vi "InitDrivebase.vi"   [LabVIEW 2020]
doc: "This VI initializes devices related directly to the drive subsystem."
uses:
  <vilib>/Rock Robotics/WPI/Solenoid/WPI_SolenoidChannel.ctl
  <vilib>/Rock Robotics/WPI/ThirdParty/Phoenix-LabVIEW/Motor Controller/Controls/CTRE_Phoenix_MotorControl_NeutralMode.ctl
  <vilib>/Rock Robotics/WPI/ThirdParty/Phoenix-LabVIEW/Motor Controller/Controls/CTRE_Phoenix_MotorControl_SupplyCurrentLimitConfiguration.ctl
  <vilib>/Rock Robotics/WPI/ThirdParty/Phoenix-LabVIEW/Motor Controller/Controls/CTRE_Phoenix_MotorControl_FeedbackDevice_TalonFX.ctl
  <vilib>/Rock Robotics/WPI/ThirdParty/Phoenix-LabVIEW/Motor Controller/Controls/CTRE_Phoenix_MotorControl_TalonFXInvertType.ctl
  <vilib>/Rock Robotics/WPI/Solenoid/WPI_SolenoidOpenDouble.vi
  refnums.vi
types:
  T1 = typedef "WPI_SolenoidChannel.ctl" = enum8{"Solenoid 0", "Solenoid 1", "Solenoid 2", "Solenoid 3", "Solenoid 4", "Solenoid 5", "Solenoid 6", "Solenoid 7", "Solenoid 8", "Solenoid 9", "Solenoid 10", "Solenoid 11", "Solenoid 12", "Solenoid 13", "Solenoid 14", "Solenoid 15", "Invalid"}
  T2 = typedef "CTRE_Phoenix_MotorControl_TalonFXInvertType.ctl" = enum16{"Counter-Clockwise", "Clockwise"}
  T3 = typedef "CTRE_Phoenix_MotorControl_FeedbackDevice_TalonFX.ctl" = i8
  T4 = typedef "CTRE_Phoenix_MotorControl_SupplyCurrentLimitConfiguration.ctl" = cluster{"Enable?":bool, "Current Limit":dbl, "Threshold Current":dbl, "Threshold Time":dbl}
  T5 = typedef "CTRE_Phoenix_MotorControl_NeutralMode.ctl" = enum8{"EEPROMSetting", "Override to Coast", "Override to Brake"}
  T6 = typedef "WPI_MotorControlDeviceRef.ctl" = cluster{"DeviceStatus":errorcluster, "Type":T7, "PWM":cluster{"PWM Channel":T8, "DeadBand":T9}, "CAN":cluster{"Device Number":u8, "SetOutput VI Ref":variant, "GetOutput VI Ref":variant, "Enable VI Ref":variant, "Disable VI Ref":variant, "Data":variant}, "Invert":bool, "DIO PWM":cluster{"PWM \"Enable\" Channel":T8, "DIOChannel":T10, "PWM Rate":dbl}}
  T7 = typedef "WPI_MotorControlType.ctl" = enum16{"PWM", "CAN", "DIO PWM"}
  T8 = typedef "FPGA_DIOPWMChannel.ctl" = enum8{"PWM 0", "PWM 1", "PWM 2", "PWM 3", "PWM 4", "PWM 5", "PWM 6", "PWM 7", "PWM 8", "PWM 9", "PWM MXP 0", "PWM MXP 1", "PWM MXP 2", "PWM MXP 3", "PWM MXP 4", "PWM MXP 5", "PWM MXP 6", "PWM MXP 7", "PWM MXP 8", "PWM MXP 9", "Invalid"}
  T9 = typedef "WPI_PWMDeadband.ctl" = cluster{"Name":string, "maxPositivePwm":i32, "minPositivePwm":i32, "centerPwm":i32, "maxNegativePwm":i32, "minNegativePwm":i32, "angularRange":u16}
  T10 = typedef "FPGA_DIOChannel.ctl" = enum8{"DIO 0", "DIO 1", "DIO 2", "DIO 3", "DIO 4", "DIO 5", "DIO 6", "DIO 7", "DIO 8", "DIO 9", "DIO MXP 0", "DIO MXP 1", "DIO MXP 2", "DIO MXP 3", "DIO MXP 4", "DIO MXP 5", "DIO MXP 6", "DIO MXP 7", "DIO MXP 8", "DIO MXP 9", "DIO MXP 10", "DIO MXP 11", "DIO MXP 12", "DIO MXP 13", "DIO MXP 14", "DIO MXP 15", "SPI Port CS1", "SPI Port CS2", "SPI Port CS3", "SPI Port MISO", "SPI Port MOSI", "Invalid"}
  T11 = typedef "WPI_SolenoidDevRef.ctl" = cluster{"DevStatus":errorcluster, "Pneumatics Control Module":u8, "Forward Solenoid Channel":T1, "Reverse Solenoid Channel":T1}
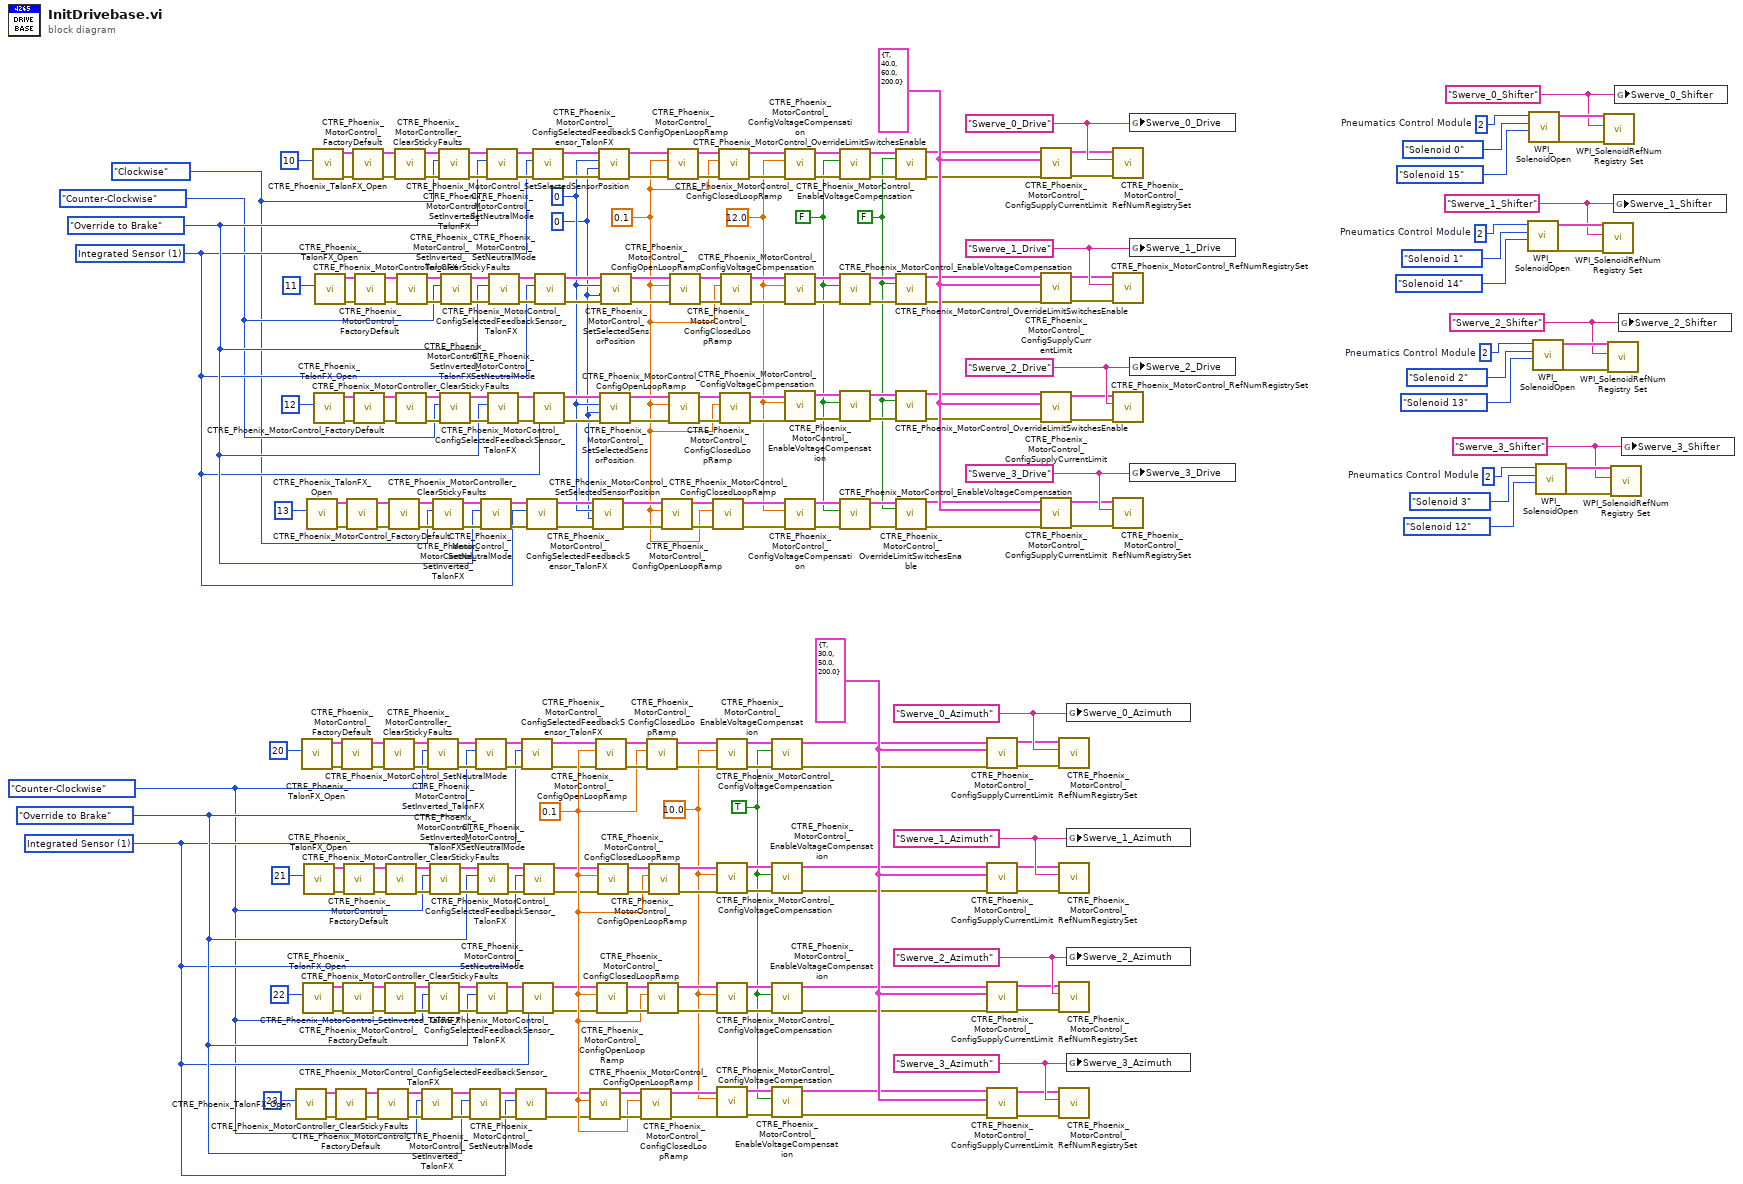
[diagram p0: block diagram]
diagram:
  w9 = FALSE ("Override Limit Switch Enable?")
  w27 = "Swerve_0_Shifter" ("refnum name")
  w32 = u8 2  # Pneumatics Control Module
  w33 = "Swerve_1_Shifter" ("refnum name")
  w38 = u8 2  # Pneumatics Control Module
  w39 = "Swerve_2_Shifter" ("refnum name")
  w44 = u8 2  # Pneumatics Control Module
  w45 = CTRE_Phoenix_MotorControl_TalonFXInvertType."Clockwise" ("Invert Type")
  w47 = TRUE ("Enable Voltage Compensation?")
  w48 = 10.0 ("Saturation Voltage")
  w49 = FALSE ("Enable Voltage Compensation?")
  w50 = 12.0 ("Saturation Voltage")
  w91 = T3 1 items=["Integrated Sensor"=1, "Sensor Sum (S0 + S1)"=9, "Sensor Difference (D0 - D1)"=10, "Remote Source 0"=11, "Remote Source 1"=12, "None"=14, "Software Emulated"=15] ("Talon FX Feedback Device")
  w94 = T4 {"Enable?"=TRUE, "Current Limit"=30.0, "Threshold Current"=50.0, "Threshold Time"=200.0} ("Supply Current Limit Configuration")
  w92 = 0.1 ("secondsFromNeutralToFull")
  w93 = CTRE_Phoenix_MotorControl_NeutralMode."Override to Brake" ("Motor Control Neutral Mode")
  w26 = CTRE_Phoenix_MotorControl_TalonFXInvertType."Counter-Clockwise" ("Invert Type")
  w108 = "Swerve_0_Azimuth" ("refnum name")
  w124 = "Swerve_1_Azimuth" ("refnum name")
  w140 = "Swerve_2_Azimuth" ("refnum name")
  w156 = "Swerve_3_Azimuth" ("refnum name")
  w162 = T3 1 items=["Integrated Sensor"=1, "Sensor Sum (S0 + S1)"=9, "Sensor Difference (D0 - D1)"=10, "Remote Source 0"=11, "Remote Source 1"=12, "None"=14, "Software Emulated"=15] ("Talon FX Feedback Device")
  w164 = T4 {"Enable?"=TRUE, "Current Limit"=40.0, "Threshold Current"=60.0, "Threshold Time"=200.0} ("Supply Current Limit Configuration")
  w159 = 0.1 ("secondsFromNeutralToFull")
  w160 = u32 0 ("pidLoopIdx")
  w161 = 0 ("New Sensor Position")
  w163 = CTRE_Phoenix_MotorControl_NeutralMode."Override to Brake" ("Motor Control Neutral Mode")
  w46 = CTRE_Phoenix_MotorControl_TalonFXInvertType."Counter-Clockwise" ("Invert Type")
  w180 = "Swerve_0_Drive" ("refnum name")
  w200 = "Swerve_1_Drive" ("refnum name")
  w220 = "Swerve_2_Drive" ("refnum name")
  w240 = "Swerve_3_Drive" ("refnum name")
  w245 = "Swerve_3_Shifter" ("refnum name")
  w250 = u8 2  # Pneumatics Control Module
  n1 = call <vilib>:"CTRE_Phoenix_TalonFX_Open.vi"("Device Number"=u8 23 ("Drive 4L")) -> ("error out"=w145:errorcluster, "PhoenixMotorControlDevRef"=w152:T6)  [unwired: 9 in]
  n2 = call <vilib>:"CTRE_Phoenix_TalonFX_Open.vi"("Device Number"=u8 20 ("Drive 4L")) -> ("error out"=w97:errorcluster, "PhoenixMotorControlDevRef"=w104:T6)  [unwired: 9 in]
  n3 = call <vilib>:"CTRE_Phoenix_TalonFX_Open.vi"("Device Number"=u8 22 ("Drive 4L")) -> ("error out"=w129:errorcluster, "PhoenixMotorControlDevRef"=w136:T6)  [unwired: 9 in]
  n4 = call <vilib>:"CTRE_Phoenix_TalonFX_Open.vi"("Device Number"=u8 21 ("Drive 4L")) -> ("error out"=w113:errorcluster, "PhoenixMotorControlDevRef"=w120:T6)  [unwired: 9 in]
  n5 = call <vilib>:"CTRE_Phoenix_TalonFX_Open.vi"("Device Number"=u8 13 ("Drive 4L")) -> ("error out"=w229:errorcluster, "PhoenixMotorControlDevRef"=w236:T6)  [unwired: 9 in]
  n6 = call <vilib>:"CTRE_Phoenix_TalonFX_Open.vi"("Device Number"=u8 10 ("Drive 4L")) -> ("error out"=w169:errorcluster, "PhoenixMotorControlDevRef"=w176:T6)  [unwired: 9 in]
  n7 = call <vilib>:"CTRE_Phoenix_TalonFX_Open.vi"("Device Number"=u8 12 ("Drive 4L")) -> ("error out"=w209:errorcluster, "PhoenixMotorControlDevRef"=w216:T6)  [unwired: 9 in]
  n8 = call <vilib>:"CTRE_Phoenix_TalonFX_Open.vi"("Device Number"=u8 11 ("Drive 4L")) -> ("error out"=w189:errorcluster, "PhoenixMotorControlDevRef"=w196:T6)  [unwired: 9 in]
  n9 = call <vilib>:"CTRE_Phoenix_MotorControl_FactoryDefault.vi"("error in"=w145, "PhoenixMotorControlDevRef"=w152) -> ("error out"=w148:errorcluster, "PhoenixMotorControlDevRef"=w149:T6)  [unwired: 8 in]
  n10 = call <vilib>:"CTRE_Phoenix_MotorControl_FactoryDefault.vi"("error in"=w97, "PhoenixMotorControlDevRef"=w104) -> ("error out"=w100:errorcluster, "PhoenixMotorControlDevRef"=w101:T6)  [unwired: 8 in]
  n11 = call <vilib>:"CTRE_Phoenix_MotorControl_FactoryDefault.vi"("error in"=w129, "PhoenixMotorControlDevRef"=w136) -> ("error out"=w132:errorcluster, "PhoenixMotorControlDevRef"=w133:T6)  [unwired: 8 in]
  n12 = call <vilib>:"CTRE_Phoenix_MotorControl_FactoryDefault.vi"("error in"=w113, "PhoenixMotorControlDevRef"=w120) -> ("error out"=w116:errorcluster, "PhoenixMotorControlDevRef"=w117:T6)  [unwired: 8 in]
  n13 = call <vilib>:"CTRE_Phoenix_MotorControl_FactoryDefault.vi"("error in"=w229, "PhoenixMotorControlDevRef"=w236) -> ("error out"=w232:errorcluster, "PhoenixMotorControlDevRef"=w233:T6)  [unwired: 8 in]
  n14 = call <vilib>:"CTRE_Phoenix_MotorControl_FactoryDefault.vi"("error in"=w169, "PhoenixMotorControlDevRef"=w176) -> ("error out"=w172:errorcluster, "PhoenixMotorControlDevRef"=w173:T6)  [unwired: 8 in]
  n15 = call <vilib>:"CTRE_Phoenix_MotorControl_FactoryDefault.vi"("error in"=w209, "PhoenixMotorControlDevRef"=w216) -> ("error out"=w212:errorcluster, "PhoenixMotorControlDevRef"=w213:T6)  [unwired: 8 in]
  n16 = call <vilib>:"CTRE_Phoenix_MotorControl_FactoryDefault.vi"("error in"=w189, "PhoenixMotorControlDevRef"=w196) -> ("error out"=w192:errorcluster, "PhoenixMotorControlDevRef"=w193:T6)  [unwired: 8 in]
  n17 = call <vilib>:"CTRE_Phoenix_MotorController_ClearStickyFaults.vi"("error in"=w148, "PhoenixMotorControlDevRef"=w149) -> ("error out"=w147:errorcluster, "PhoenixMotorControlDevRef"=w146:T6)  [unwired: 8 in]
  n18 = call <vilib>:"CTRE_Phoenix_MotorController_ClearStickyFaults.vi"("error in"=w100, "PhoenixMotorControlDevRef"=w101) -> ("error out"=w99:errorcluster, "PhoenixMotorControlDevRef"=w98:T6)  [unwired: 8 in]
  n19 = call <vilib>:"CTRE_Phoenix_MotorController_ClearStickyFaults.vi"("error in"=w132, "PhoenixMotorControlDevRef"=w133) -> ("error out"=w131:errorcluster, "PhoenixMotorControlDevRef"=w130:T6)  [unwired: 8 in]
  n20 = call <vilib>:"CTRE_Phoenix_MotorController_ClearStickyFaults.vi"("error in"=w116, "PhoenixMotorControlDevRef"=w117) -> ("error out"=w115:errorcluster, "PhoenixMotorControlDevRef"=w114:T6)  [unwired: 8 in]
  n21 = call <vilib>:"CTRE_Phoenix_MotorController_ClearStickyFaults.vi"("error in"=w232, "PhoenixMotorControlDevRef"=w233) -> ("error out"=w231:errorcluster, "PhoenixMotorControlDevRef"=w230:T6)  [unwired: 8 in]
  n22 = call <vilib>:"CTRE_Phoenix_MotorController_ClearStickyFaults.vi"("error in"=w172, "PhoenixMotorControlDevRef"=w173) -> ("error out"=w171:errorcluster, "PhoenixMotorControlDevRef"=w170:T6)  [unwired: 8 in]
  n23 = call <vilib>:"CTRE_Phoenix_MotorController_ClearStickyFaults.vi"("error in"=w212, "PhoenixMotorControlDevRef"=w213) -> ("error out"=w211:errorcluster, "PhoenixMotorControlDevRef"=w210:T6)  [unwired: 8 in]
  n24 = call <vilib>:"CTRE_Phoenix_MotorController_ClearStickyFaults.vi"("error in"=w192, "PhoenixMotorControlDevRef"=w193) -> ("error out"=w191:errorcluster, "PhoenixMotorControlDevRef"=w190:T6)  [unwired: 8 in]
  n25 = call <vilib>:"CTRE_Phoenix_MotorControl_SetInverted_TalonFX.vi"("error in (no error)"=w147, "Invert Type"=w26, "PhoenixMotorControlDevRef"=w146) -> ("error out"=w157:errorcluster, "PhoenixMotorControlDevRef"=w158:T6)  [unwired: 7 in]
  n26 = call <vilib>:"CTRE_Phoenix_MotorControl_SetInverted_TalonFX.vi"("error in (no error)"=w99, "Invert Type"=w26, "PhoenixMotorControlDevRef"=w98) -> ("error out"=w109:errorcluster, "PhoenixMotorControlDevRef"=w110:T6)  [unwired: 7 in]
  n27 = call <vilib>:"CTRE_Phoenix_MotorControl_SetInverted_TalonFX.vi"("error in (no error)"=w131, "Invert Type"=w26, "PhoenixMotorControlDevRef"=w130) -> ("error out"=w141:errorcluster, "PhoenixMotorControlDevRef"=w142:T6)  [unwired: 7 in]
  n28 = call <vilib>:"CTRE_Phoenix_MotorControl_SetInverted_TalonFX.vi"("error in (no error)"=w115, "Invert Type"=w26, "PhoenixMotorControlDevRef"=w114) -> ("error out"=w125:errorcluster, "PhoenixMotorControlDevRef"=w126:T6)  [unwired: 7 in]
  n29 = call <vilib>:"CTRE_Phoenix_MotorControl_SetInverted_TalonFX.vi"("error in (no error)"=w231, "Invert Type"=w45, "PhoenixMotorControlDevRef"=w230) -> ("error out"=w243:errorcluster, "PhoenixMotorControlDevRef"=w244:T6)  [unwired: 7 in]
  n30 = call <vilib>:"CTRE_Phoenix_MotorControl_SetInverted_TalonFX.vi"("error in (no error)"=w171, "Invert Type"=w45, "PhoenixMotorControlDevRef"=w170) -> ("error out"=w183:errorcluster, "PhoenixMotorControlDevRef"=w184:T6)  [unwired: 7 in]
  n31 = call <vilib>:"CTRE_Phoenix_MotorControl_SetInverted_TalonFX.vi"("error in (no error)"=w211, "Invert Type"=w46, "PhoenixMotorControlDevRef"=w210) -> ("error out"=w223:errorcluster, "PhoenixMotorControlDevRef"=w224:T6)  [unwired: 7 in]
  n32 = call <vilib>:"CTRE_Phoenix_MotorControl_SetInverted_TalonFX.vi"("error in (no error)"=w191, "Invert Type"=w46, "PhoenixMotorControlDevRef"=w190) -> ("error out"=w203:errorcluster, "PhoenixMotorControlDevRef"=w204:T6)  [unwired: 7 in]
  n33 = call <vilib>:"CTRE_Phoenix_MotorControl_SetNeutralMode.vi"("error in (no error)"=w157, "Motor Control Neutral Mode"=w93, "PhoenixMotorControlDevRef"=w158) -> ("error out"=w143:errorcluster, "PhoenixMotorControlDevRef"=w144:T6)  [unwired: 7 in]
  n34 = call <vilib>:"CTRE_Phoenix_MotorControl_SetNeutralMode.vi"("error in (no error)"=w109, "Motor Control Neutral Mode"=w93, "PhoenixMotorControlDevRef"=w110) -> ("error out"=w95:errorcluster, "PhoenixMotorControlDevRef"=w96:T6)  [unwired: 7 in]
  n35 = call <vilib>:"CTRE_Phoenix_MotorControl_SetNeutralMode.vi"("error in (no error)"=w141, "Motor Control Neutral Mode"=w93, "PhoenixMotorControlDevRef"=w142) -> ("error out"=w127:errorcluster, "PhoenixMotorControlDevRef"=w128:T6)  [unwired: 7 in]
  n36 = call <vilib>:"CTRE_Phoenix_MotorControl_SetNeutralMode.vi"("error in (no error)"=w125, "Motor Control Neutral Mode"=w93, "PhoenixMotorControlDevRef"=w126) -> ("error out"=w111:errorcluster, "PhoenixMotorControlDevRef"=w112:T6)  [unwired: 7 in]
  n37 = call <vilib>:"CTRE_Phoenix_MotorControl_SetNeutralMode.vi"("error in (no error)"=w243, "Motor Control Neutral Mode"=w163, "PhoenixMotorControlDevRef"=w244) -> ("error out"=w227:errorcluster, "PhoenixMotorControlDevRef"=w228:T6)  [unwired: 7 in]
  n38 = call <vilib>:"CTRE_Phoenix_MotorControl_SetNeutralMode.vi"("error in (no error)"=w183, "Motor Control Neutral Mode"=w163, "PhoenixMotorControlDevRef"=w184) -> ("error out"=w167:errorcluster, "PhoenixMotorControlDevRef"=w168:T6)  [unwired: 7 in]
  n39 = call <vilib>:"CTRE_Phoenix_MotorControl_SetNeutralMode.vi"("error in (no error)"=w223, "Motor Control Neutral Mode"=w163, "PhoenixMotorControlDevRef"=w224) -> ("error out"=w207:errorcluster, "PhoenixMotorControlDevRef"=w208:T6)  [unwired: 7 in]
  n40 = call <vilib>:"CTRE_Phoenix_MotorControl_SetNeutralMode.vi"("error in (no error)"=w203, "Motor Control Neutral Mode"=w163, "PhoenixMotorControlDevRef"=w204) -> ("error out"=w187:errorcluster, "PhoenixMotorControlDevRef"=w188:T6)  [unwired: 7 in]
  n41 = call <vilib>:"CTRE_Phoenix_MotorControl_ConfigSelectedFeedbackSensor_TalonFX.vi"("error in (no error)"=w143, "Talon FX Feedback Device"=w91, "PhoenixMotorControlDevRef"=w144) -> ("error out"=w7:errorcluster, "PhoenixMotorControlDevRef"=w8:T6)  [unwired: 7 in]
  n42 = call <vilib>:"CTRE_Phoenix_MotorControl_ConfigSelectedFeedbackSensor_TalonFX.vi"("error in (no error)"=w95, "Talon FX Feedback Device"=w91, "PhoenixMotorControlDevRef"=w96) -> ("error out"=w1:errorcluster, "PhoenixMotorControlDevRef"=w2:T6)  [unwired: 7 in]
  n43 = call <vilib>:"CTRE_Phoenix_MotorControl_ConfigSelectedFeedbackSensor_TalonFX.vi"("error in (no error)"=w127, "Talon FX Feedback Device"=w91, "PhoenixMotorControlDevRef"=w128) -> ("error out"=w5:errorcluster, "PhoenixMotorControlDevRef"=w6:T6)  [unwired: 7 in]
  n44 = call <vilib>:"CTRE_Phoenix_MotorControl_ConfigSelectedFeedbackSensor_TalonFX.vi"("error in (no error)"=w111, "Talon FX Feedback Device"=w91, "PhoenixMotorControlDevRef"=w112) -> ("error out"=w3:errorcluster, "PhoenixMotorControlDevRef"=w4:T6)  [unwired: 7 in]
  n45 = call <vilib>:"CTRE_Phoenix_MotorControl_ConfigSelectedFeedbackSensor_TalonFX.vi"("error in (no error)"=w227, "Talon FX Feedback Device"=w162, "PhoenixMotorControlDevRef"=w228) -> ("error out"=w225:errorcluster, "PhoenixMotorControlDevRef"=w226:T6)  [unwired: 7 in]
  n46 = call <vilib>:"CTRE_Phoenix_MotorControl_ConfigSelectedFeedbackSensor_TalonFX.vi"("error in (no error)"=w167, "Talon FX Feedback Device"=w162, "PhoenixMotorControlDevRef"=w168) -> ("error out"=w165:errorcluster, "PhoenixMotorControlDevRef"=w166:T6)  [unwired: 7 in]
  n47 = call <vilib>:"CTRE_Phoenix_MotorControl_ConfigSelectedFeedbackSensor_TalonFX.vi"("error in (no error)"=w207, "Talon FX Feedback Device"=w162, "PhoenixMotorControlDevRef"=w208) -> ("error out"=w205:errorcluster, "PhoenixMotorControlDevRef"=w206:T6)  [unwired: 7 in]
  n48 = call <vilib>:"CTRE_Phoenix_MotorControl_ConfigSelectedFeedbackSensor_TalonFX.vi"("error in (no error)"=w187, "Talon FX Feedback Device"=w162, "PhoenixMotorControlDevRef"=w188) -> ("error out"=w185:errorcluster, "PhoenixMotorControlDevRef"=w186:T6)  [unwired: 7 in]
  n49 = call <vilib>:"CTRE_Phoenix_MotorControl_ConfigOpenLoopRamp.vi"("error in (no error)"=w7, "secondsFromNeutralToFull"=w92, "PhoenixMotorControlDevRef"=w8) -> ("error out"=w150:errorcluster, "PhoenixMotorControlDevRef"=w151:T6)  [unwired: 7 in]
  n50 = call <vilib>:"CTRE_Phoenix_MotorControl_SetSelectedSensorPosition.vi"("error in (no error)"=w225, "pidLoopIdx"=w160, "New Sensor Position"=w161, "PhoenixMotorControlDevRef"=w226) -> ("error out"=w242:errorcluster, "PhoenixMotorControlDevRef"=w241:T6)  [unwired: 6 in]
  n51 = call <vilib>:"CTRE_Phoenix_MotorControl_ConfigOpenLoopRamp.vi"("error in (no error)"=w1, "secondsFromNeutralToFull"=w92, "PhoenixMotorControlDevRef"=w2) -> ("error out"=w102:errorcluster, "PhoenixMotorControlDevRef"=w103:T6)  [unwired: 7 in]
  n52 = call <vilib>:"CTRE_Phoenix_MotorControl_ConfigOpenLoopRamp.vi"("error in (no error)"=w5, "secondsFromNeutralToFull"=w92, "PhoenixMotorControlDevRef"=w6) -> ("error out"=w134:errorcluster, "PhoenixMotorControlDevRef"=w135:T6)  [unwired: 7 in]
  n53 = call <vilib>:"CTRE_Phoenix_MotorControl_ConfigOpenLoopRamp.vi"("error in (no error)"=w3, "secondsFromNeutralToFull"=w92, "PhoenixMotorControlDevRef"=w4) -> ("error out"=w118:errorcluster, "PhoenixMotorControlDevRef"=w119:T6)  [unwired: 7 in]
  n54 = call <vilib>:"CTRE_Phoenix_MotorControl_SetSelectedSensorPosition.vi"("error in (no error)"=w165, "pidLoopIdx"=w160, "New Sensor Position"=w161, "PhoenixMotorControlDevRef"=w166) -> ("error out"=w182:errorcluster, "PhoenixMotorControlDevRef"=w181:T6)  [unwired: 6 in]
  n55 = call <vilib>:"CTRE_Phoenix_MotorControl_SetSelectedSensorPosition.vi"("error in (no error)"=w205, "pidLoopIdx"=w160, "New Sensor Position"=w161, "PhoenixMotorControlDevRef"=w206) -> ("error out"=w222:errorcluster, "PhoenixMotorControlDevRef"=w221:T6)  [unwired: 6 in]
  n56 = call <vilib>:"CTRE_Phoenix_MotorControl_SetSelectedSensorPosition.vi"("error in (no error)"=w185, "pidLoopIdx"=w160, "New Sensor Position"=w161, "PhoenixMotorControlDevRef"=w186) -> ("error out"=w202:errorcluster, "PhoenixMotorControlDevRef"=w201:T6)  [unwired: 6 in]
  n57 = call <vilib>:"CTRE_Phoenix_MotorControl_ConfigClosedLoopRamp.vi"("error in (no error)"=w150, "secondsFromNeutralToFull"=w92, "PhoenixMotorControlDevRef"=w151) -> ("error out"=w53:errorcluster, "PhoenixMotorControlDevRef"=w54:T6)  [unwired: 7 in]
  n58 = call <vilib>:"CTRE_Phoenix_MotorControl_ConfigClosedLoopRamp.vi"("error in (no error)"=w102, "secondsFromNeutralToFull"=w92, "PhoenixMotorControlDevRef"=w103) -> ("error out"=w65:errorcluster, "PhoenixMotorControlDevRef"=w66:T6)  [unwired: 7 in]
  n59 = call <vilib>:"CTRE_Phoenix_MotorControl_ConfigClosedLoopRamp.vi"("error in (no error)"=w134, "secondsFromNeutralToFull"=w92, "PhoenixMotorControlDevRef"=w135) -> ("error out"=w57:errorcluster, "PhoenixMotorControlDevRef"=w58:T6)  [unwired: 7 in]
  n60 = call <vilib>:"CTRE_Phoenix_MotorControl_ConfigClosedLoopRamp.vi"("error in (no error)"=w118, "secondsFromNeutralToFull"=w92, "PhoenixMotorControlDevRef"=w119) -> ("error out"=w61:errorcluster, "PhoenixMotorControlDevRef"=w62:T6)  [unwired: 7 in]
  n61 = call <vilib>:"CTRE_Phoenix_MotorControl_ConfigOpenLoopRamp.vi"("error in (no error)"=w242, "secondsFromNeutralToFull"=w159, "PhoenixMotorControlDevRef"=w241) -> ("error out"=w234:errorcluster, "PhoenixMotorControlDevRef"=w235:T6)  [unwired: 7 in]
  n62 = call <vilib>:"CTRE_Phoenix_MotorControl_ConfigOpenLoopRamp.vi"("error in (no error)"=w182, "secondsFromNeutralToFull"=w159, "PhoenixMotorControlDevRef"=w181) -> ("error out"=w174:errorcluster, "PhoenixMotorControlDevRef"=w175:T6)  [unwired: 7 in]
  n63 = call <vilib>:"CTRE_Phoenix_MotorControl_ConfigOpenLoopRamp.vi"("error in (no error)"=w222, "secondsFromNeutralToFull"=w159, "PhoenixMotorControlDevRef"=w221) -> ("error out"=w214:errorcluster, "PhoenixMotorControlDevRef"=w215:T6)  [unwired: 7 in]
  n64 = call <vilib>:"CTRE_Phoenix_MotorControl_ConfigOpenLoopRamp.vi"("error in (no error)"=w202, "secondsFromNeutralToFull"=w159, "PhoenixMotorControlDevRef"=w201) -> ("error out"=w194:errorcluster, "PhoenixMotorControlDevRef"=w195:T6)  [unwired: 7 in]
  n65 = call <vilib>:"CTRE_Phoenix_MotorControl_ConfigClosedLoopRamp.vi"("error in (no error)"=w234, "secondsFromNeutralToFull"=w159, "PhoenixMotorControlDevRef"=w235) -> ("error out"=w67:errorcluster, "PhoenixMotorControlDevRef"=w68:T6)  [unwired: 7 in]
  n66 = call <vilib>:"CTRE_Phoenix_MotorControl_ConfigVoltageCompensation.vi"("error in (no error)"=w65, "Saturation Voltage"=w48, "PhoenixMotorControlDevRef"=w66) -> ("error out"=w81:errorcluster, "PhoenixMotorControlDevRef"=w82:T6)  [unwired: 7 in]
  n67 = call <vilib>:"CTRE_Phoenix_MotorControl_ConfigVoltageCompensation.vi"("error in (no error)"=w61, "Saturation Voltage"=w48, "PhoenixMotorControlDevRef"=w62) -> ("error out"=w79:errorcluster, "PhoenixMotorControlDevRef"=w80:T6)  [unwired: 7 in]
  n68 = call <vilib>:"CTRE_Phoenix_MotorControl_ConfigVoltageCompensation.vi"("error in (no error)"=w57, "Saturation Voltage"=w48, "PhoenixMotorControlDevRef"=w58) -> ("error out"=w77:errorcluster, "PhoenixMotorControlDevRef"=w78:T6)  [unwired: 7 in]
  n69 = call <vilib>:"CTRE_Phoenix_MotorControl_ConfigVoltageCompensation.vi"("error in (no error)"=w53, "Saturation Voltage"=w48, "PhoenixMotorControlDevRef"=w54) -> ("error out"=w75:errorcluster, "PhoenixMotorControlDevRef"=w76:T6)  [unwired: 7 in]
  n70 = call <vilib>:"CTRE_Phoenix_MotorControl_ConfigClosedLoopRamp.vi"("error in (no error)"=w174, "secondsFromNeutralToFull"=w159, "PhoenixMotorControlDevRef"=w175) -> ("error out"=w73:errorcluster, "PhoenixMotorControlDevRef"=w74:T6)  [unwired: 7 in]
  n71 = call <vilib>:"CTRE_Phoenix_MotorControl_ConfigClosedLoopRamp.vi"("error in (no error)"=w214, "secondsFromNeutralToFull"=w159, "PhoenixMotorControlDevRef"=w215) -> ("error out"=w69:errorcluster, "PhoenixMotorControlDevRef"=w70:T6)  [unwired: 7 in]
  n72 = call <vilib>:"CTRE_Phoenix_MotorControl_ConfigClosedLoopRamp.vi"("error in (no error)"=w194, "secondsFromNeutralToFull"=w159, "PhoenixMotorControlDevRef"=w195) -> ("error out"=w71:errorcluster, "PhoenixMotorControlDevRef"=w72:T6)  [unwired: 7 in]
  n73 = call <vilib>:"CTRE_Phoenix_MotorControl_EnableVoltageCompensation.vi"("error in (no error)"=w81, "Enable Voltage Compensation?"=w47, "PhoenixMotorControlDevRef"=w82) -> ("error out"=w63:errorcluster, "PhoenixMotorControlDevRef"=w64:T6)  [unwired: 7 in]
  n74 = call <vilib>:"CTRE_Phoenix_MotorControl_EnableVoltageCompensation.vi"("error in (no error)"=w79, "Enable Voltage Compensation?"=w47, "PhoenixMotorControlDevRef"=w80) -> ("error out"=w59:errorcluster, "PhoenixMotorControlDevRef"=w60:T6)  [unwired: 7 in]
  n75 = call <vilib>:"CTRE_Phoenix_MotorControl_EnableVoltageCompensation.vi"("error in (no error)"=w77, "Enable Voltage Compensation?"=w47, "PhoenixMotorControlDevRef"=w78) -> ("error out"=w55:errorcluster, "PhoenixMotorControlDevRef"=w56:T6)  [unwired: 7 in]
  n76 = call <vilib>:"CTRE_Phoenix_MotorControl_EnableVoltageCompensation.vi"("error in (no error)"=w75, "Enable Voltage Compensation?"=w47, "PhoenixMotorControlDevRef"=w76) -> ("error out"=w51:errorcluster, "PhoenixMotorControlDevRef"=w52:T6)  [unwired: 7 in]
  n77 = call <vilib>:"CTRE_Phoenix_MotorControl_ConfigVoltageCompensation.vi"("error in (no error)"=w73, "Saturation Voltage"=w50, "PhoenixMotorControlDevRef"=w74) -> ("error out"=w89:errorcluster, "PhoenixMotorControlDevRef"=w90:T6)  [unwired: 7 in]
  n78 = call <vilib>:"CTRE_Phoenix_MotorControl_ConfigVoltageCompensation.vi"("error in (no error)"=w71, "Saturation Voltage"=w50, "PhoenixMotorControlDevRef"=w72) -> ("error out"=w87:errorcluster, "PhoenixMotorControlDevRef"=w88:T6)  [unwired: 7 in]
  n79 = call <vilib>:"CTRE_Phoenix_MotorControl_ConfigVoltageCompensation.vi"("error in (no error)"=w69, "Saturation Voltage"=w50, "PhoenixMotorControlDevRef"=w70) -> ("error out"=w85:errorcluster, "PhoenixMotorControlDevRef"=w86:T6)  [unwired: 7 in]
  n80 = call <vilib>:"CTRE_Phoenix_MotorControl_ConfigVoltageCompensation.vi"("error in (no error)"=w67, "Saturation Voltage"=w50, "PhoenixMotorControlDevRef"=w68) -> ("error out"=w83:errorcluster, "PhoenixMotorControlDevRef"=w84:T6)  [unwired: 7 in]
  n81 = call <vilib>:"CTRE_Phoenix_MotorControl_EnableVoltageCompensation.vi"("error in (no error)"=w89, "Enable Voltage Compensation?"=w49, "PhoenixMotorControlDevRef"=w90) -> ("error out"=w24:errorcluster, "PhoenixMotorControlDevRef"=w25:T6)  [unwired: 7 in]
  n82 = call <vilib>:"CTRE_Phoenix_MotorControl_EnableVoltageCompensation.vi"("error in (no error)"=w87, "Enable Voltage Compensation?"=w49, "PhoenixMotorControlDevRef"=w88) -> ("error out"=w22:errorcluster, "PhoenixMotorControlDevRef"=w23:T6)  [unwired: 7 in]
  n83 = call <vilib>:"CTRE_Phoenix_MotorControl_EnableVoltageCompensation.vi"("error in (no error)"=w85, "Enable Voltage Compensation?"=w49, "PhoenixMotorControlDevRef"=w86) -> ("error out"=w20:errorcluster, "PhoenixMotorControlDevRef"=w21:T6)  [unwired: 7 in]
  n84 = call <vilib>:"CTRE_Phoenix_MotorControl_EnableVoltageCompensation.vi"("error in (no error)"=w83, "Enable Voltage Compensation?"=w49, "PhoenixMotorControlDevRef"=w84) -> ("error out"=w18:errorcluster, "PhoenixMotorControlDevRef"=w19:T6)  [unwired: 7 in]
  n85 = call <vilib>:"CTRE_Phoenix_MotorControl_OverrideLimitSwitchesEnable.vi"("PhoenixMotorControlDevRef"=w25, "Override Limit Switch Enable?"=w9, "error in (no error)"=w24) -> ("PhoenixMotorControlDevRef"=w17:T6, "error out"=w16:errorcluster)  [unwired: 11 in]
  n86 = call <vilib>:"CTRE_Phoenix_MotorControl_OverrideLimitSwitchesEnable.vi"("PhoenixMotorControlDevRef"=w23, "Override Limit Switch Enable?"=w9, "error in (no error)"=w22) -> ("PhoenixMotorControlDevRef"=w15:T6, "error out"=w14:errorcluster)  [unwired: 11 in]
  n87 = call <vilib>:"CTRE_Phoenix_MotorControl_OverrideLimitSwitchesEnable.vi"("PhoenixMotorControlDevRef"=w21, "Override Limit Switch Enable?"=w9, "error in (no error)"=w20) -> ("PhoenixMotorControlDevRef"=w13:T6, "error out"=w12:errorcluster)  [unwired: 11 in]
  n88 = call <vilib>:"CTRE_Phoenix_MotorControl_OverrideLimitSwitchesEnable.vi"("PhoenixMotorControlDevRef"=w19, "Override Limit Switch Enable?"=w9, "error in (no error)"=w18) -> ("PhoenixMotorControlDevRef"=w11:T6, "error out"=w10:errorcluster)  [unwired: 11 in]
  n89 = call <vilib>:"CTRE_Phoenix_MotorControl_ConfigSupplyCurrentLimit.vi"("error in (no error)"=w63, "Supply Current Limit Configuration"=w94, "PhoenixMotorControlDevRef"=w64) -> ("error out"=w106:errorcluster, "PhoenixMotorControlDevRef"=w107:T6)  [unwired: 7 in]
  n90 = call <vilib>:"CTRE_Phoenix_MotorControl_ConfigSupplyCurrentLimit.vi"("error in (no error)"=w59, "Supply Current Limit Configuration"=w94, "PhoenixMotorControlDevRef"=w60) -> ("error out"=w122:errorcluster, "PhoenixMotorControlDevRef"=w123:T6)  [unwired: 7 in]
  n91 = call <vilib>:"CTRE_Phoenix_MotorControl_ConfigSupplyCurrentLimit.vi"("error in (no error)"=w55, "Supply Current Limit Configuration"=w94, "PhoenixMotorControlDevRef"=w56) -> ("error out"=w138:errorcluster, "PhoenixMotorControlDevRef"=w139:T6)  [unwired: 7 in]
  n92 = call <vilib>:"CTRE_Phoenix_MotorControl_ConfigSupplyCurrentLimit.vi"("error in (no error)"=w51, "Supply Current Limit Configuration"=w94, "PhoenixMotorControlDevRef"=w52) -> ("error out"=w154:errorcluster, "PhoenixMotorControlDevRef"=w155:T6)  [unwired: 7 in]
  n93 = call <vilib>:"CTRE_Phoenix_MotorControl_ConfigSupplyCurrentLimit.vi"("error in (no error)"=w16, "Supply Current Limit Configuration"=w164, "PhoenixMotorControlDevRef"=w17) -> ("error out"=w178:errorcluster, "PhoenixMotorControlDevRef"=w179:T6)  [unwired: 7 in]
  n94 = call <vilib>:"CTRE_Phoenix_MotorControl_ConfigSupplyCurrentLimit.vi"("error in (no error)"=w14, "Supply Current Limit Configuration"=w164, "PhoenixMotorControlDevRef"=w15) -> ("error out"=w198:errorcluster, "PhoenixMotorControlDevRef"=w199:T6)  [unwired: 7 in]
  n95 = call <vilib>:"CTRE_Phoenix_MotorControl_ConfigSupplyCurrentLimit.vi"("error in (no error)"=w12, "Supply Current Limit Configuration"=w164, "PhoenixMotorControlDevRef"=w13) -> ("error out"=w218:errorcluster, "PhoenixMotorControlDevRef"=w219:T6)  [unwired: 7 in]
  n96 = call <vilib>:"CTRE_Phoenix_MotorControl_ConfigSupplyCurrentLimit.vi"("error in (no error)"=w10, "Supply Current Limit Configuration"=w164, "PhoenixMotorControlDevRef"=w11) -> ("error out"=w238:errorcluster, "PhoenixMotorControlDevRef"=w239:T6)  [unwired: 7 in]
  n97 = call <vilib>:"CTRE_Phoenix_MotorControl_RefNumRegistrySet.vi"("error in (no error)"=w106, "refnum name"=w108, "PhoenixMotorControlDevRef"=w107) -> ()  [unwired: 7 in, 2 out]
  n98 = call <vilib>:"CTRE_Phoenix_MotorControl_RefNumRegistrySet.vi"("error in (no error)"=w122, "refnum name"=w124, "PhoenixMotorControlDevRef"=w123) -> ()  [unwired: 7 in, 2 out]
  n99 = call <vilib>:"CTRE_Phoenix_MotorControl_RefNumRegistrySet.vi"("error in (no error)"=w138, "refnum name"=w140, "PhoenixMotorControlDevRef"=w139) -> ()  [unwired: 7 in, 2 out]
  n100 = call <vilib>:"CTRE_Phoenix_MotorControl_RefNumRegistrySet.vi"("error in (no error)"=w154, "refnum name"=w156, "PhoenixMotorControlDevRef"=w155) -> ()  [unwired: 7 in, 2 out]
  n101 = global write "refnums.vi" "Swerve_0_Azimuth"(w108) -> ()
  n102 = global write "refnums.vi" "Swerve_1_Azimuth"(w124) -> ()
  n103 = global write "refnums.vi" "Swerve_2_Azimuth"(w140) -> ()
  n104 = global write "refnums.vi" "Swerve_3_Azimuth"(w156) -> ()
  n105 = call <vilib>:"CTRE_Phoenix_MotorControl_RefNumRegistrySet.vi"("error in (no error)"=w178, "refnum name"=w180, "PhoenixMotorControlDevRef"=w179) -> ()  [unwired: 7 in, 2 out]
  n106 = call <vilib>:"CTRE_Phoenix_MotorControl_RefNumRegistrySet.vi"("error in (no error)"=w198, "refnum name"=w200, "PhoenixMotorControlDevRef"=w199) -> ()  [unwired: 7 in, 2 out]
  n107 = call <vilib>:"CTRE_Phoenix_MotorControl_RefNumRegistrySet.vi"("error in (no error)"=w218, "refnum name"=w220, "PhoenixMotorControlDevRef"=w219) -> ()  [unwired: 7 in, 2 out]
  n108 = call <vilib>:"CTRE_Phoenix_MotorControl_RefNumRegistrySet.vi"("error in (no error)"=w238, "refnum name"=w240, "PhoenixMotorControlDevRef"=w239) -> ()  [unwired: 7 in, 2 out]
  n109 = global write "refnums.vi" "Swerve_0_Drive"(w180) -> ()
  n110 = global write "refnums.vi" "Swerve_1_Drive"(w200) -> ()
  n111 = global write "refnums.vi" "Swerve_2_Drive"(w220) -> ()
  n112 = global write "refnums.vi" "Swerve_3_Drive"(w240) -> ()
  n113 = call-poly <vilib>:"WPI_SolenoidOpen.vi"("Reverse Solenoid Channel"=WPI_SolenoidChannel."Solenoid 14", "Forward Solenoid Channel"=WPI_SolenoidChannel."Solenoid 1", "Pneumatics Device (def)"=w38) -> ("error out"=w34:errorcluster, "SolenoidDevRef"=w35:T11)  [unwired: 7 in]
  n114 = call-poly <vilib>:"WPI_SolenoidOpen.vi"("Reverse Solenoid Channel"=WPI_SolenoidChannel."Solenoid 15", "Forward Solenoid Channel"=WPI_SolenoidChannel."Solenoid 0", "Pneumatics Device (def)"=w32) -> ("error out"=w28:errorcluster, "SolenoidDevRef"=w29:T11)  [unwired: 7 in]
  n115 = call-poly <vilib>:"WPI_SolenoidOpen.vi"("Reverse Solenoid Channel"=WPI_SolenoidChannel."Solenoid 13", "Forward Solenoid Channel"=WPI_SolenoidChannel."Solenoid 2", "Pneumatics Device (def)"=w44) -> ("error out"=w40:errorcluster, "SolenoidDevRef"=w41:T11)  [unwired: 7 in]
  n116 = call-poly <vilib>:"WPI_SolenoidOpen.vi"("Reverse Solenoid Channel"=WPI_SolenoidChannel."Solenoid 12", "Forward Solenoid Channel"=WPI_SolenoidChannel."Solenoid 3", "Pneumatics Device (def)"=w250) -> ("error out"=w246:errorcluster, "SolenoidDevRef"=w247:T11)  [unwired: 7 in]
  n117 = call <vilib>:"WPI_SolenoidRefNum Registry Set.vi"("error in (no error)"=w34, "refnum name"=w33, "SolenoidDevRef"=w35) -> ()  [unwired: 7 in, 2 out]
  n118 = call <vilib>:"WPI_SolenoidRefNum Registry Set.vi"("error in (no error)"=w28, "refnum name"=w27, "SolenoidDevRef"=w29) -> ()  [unwired: 7 in, 2 out]
  n119 = call <vilib>:"WPI_SolenoidRefNum Registry Set.vi"("error in (no error)"=w40, "refnum name"=w39, "SolenoidDevRef"=w41) -> ()  [unwired: 7 in, 2 out]
  n120 = call <vilib>:"WPI_SolenoidRefNum Registry Set.vi"("error in (no error)"=w246, "refnum name"=w245, "SolenoidDevRef"=w247) -> ()  [unwired: 7 in, 2 out]
  n121 = global write "refnums.vi" "Swerve_1_Shifter"(w33) -> ()
  n122 = global write "refnums.vi" "Swerve_0_Shifter"(w27) -> ()
  n123 = global write "refnums.vi" "Swerve_2_Shifter"(w39) -> ()
  n124 = global write "refnums.vi" "Swerve_3_Shifter"(w245) -> ()
